vi "Get 2D Picture from Map.vi"(8 "error in (no error)":errorcluster, 11 "Grassfire in":refnum<class "Grassfire.lvclass">) -> (0 "error out":errorcluster, 2 "2D Picture":picture, 3 "Grassfire out":refnum<class "Grassfire.lvclass">)   [LabVIEW 2019, in "Grassfire.lvclass"]
uses:
  Grassfire.lvclass
  Grassfire.lvclass/Grassfire.ctl
  Address/Address.lvclass/Address.ctl
  Node/Node Value.lvclass/Node Value.ctl
  Node/Read Distance.vi
  Node/Read Node Type.vi
  Address/Read Row.vi
  Address/Read Column.vi
  Address/Address.lvclass
  Node/Node Value.lvclass
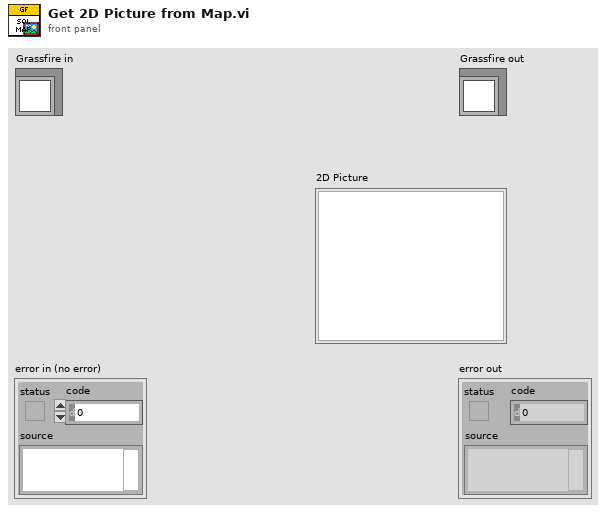
[diagram p1: front panel]
types:
  T1 = map{refnum<class "Address.lvclass">, refnum<class "Node Value.lvclass">}
  T2 = typedef "Picture Ring.lvclass/Node Type--enum.ctl" = enum16{"Empty", "Blocked", "Start", "End", "Path"}
  T3 = typedef "imagedata.ctl" = cluster{"image type":i32, "image depth":i32, "image":u8[], "mask":u8[], "colors":u32[], "Rectangle":cluster{"left":i16, "top":i16, "right":i16, "bottom":i16}}
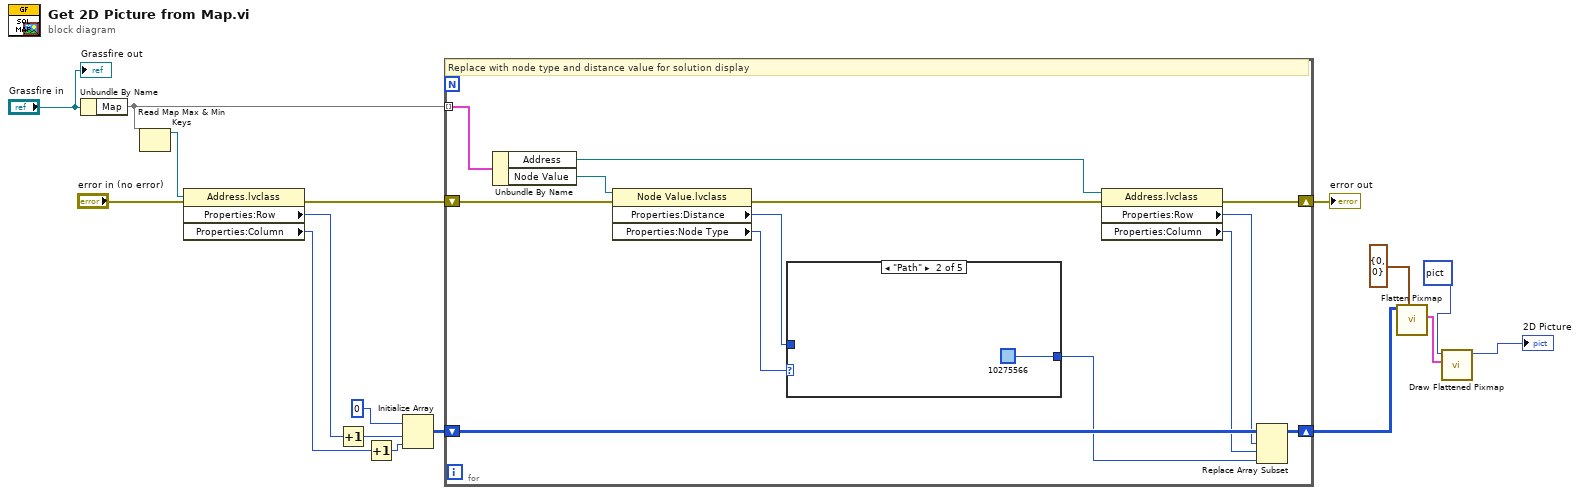
[diagram p0: block diagram]
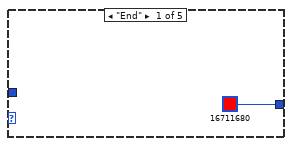
[diagram p2: hidden frame]
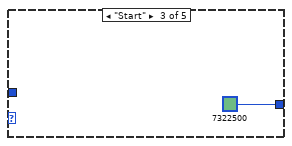
[diagram p3: hidden frame]
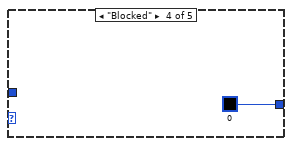
[diagram p4: hidden frame]
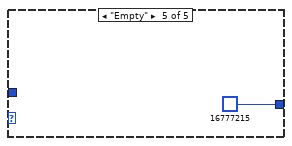
[diagram p5: hidden frame]
diagram:
  n1 = Unbundle By Name("Grassfire in") -> ("Map"=w11:T1)
  n2 = Read Map Max & Min Keys(11:w11) -> (3:w17:refnum<class "Address.lvclass">)  [unwired: 1 out]
  n3 = property class="Address.lvclass"(reference=w17, error in="error in (no error)") -> (error out=w8:errorcluster, "Properties:Row"=w16:i32, "Properties:Column"=w15:i32)  [unwired: 1 out]
  n4 = Increment(x=w16) -> (x+1=w14:i32)
  n5 = Increment(x=w15) -> (x+1=w13:i32)
  n6 = Initialize Array(u32 0, w14, w13) -> (w12:u32[][])
  n7 = for {
    shift-right: [w28] -> w2
    shift-left: w12 -> [w29]
    tunnel: w11 -> [w30] mode=indexing
    shift-right: [w21] -> w7
    shift-left: w8 -> [w23]
    # "Replace with node type and distance value for solution display"
    n8 = Unbundle By Name(w30) -> ("Address"=w27:refnum<class "Address.lvclass">, "Node Value"=w24:refnum<class "Node Value.lvclass">)
    n9 = property class="Node Value.lvclass"(reference=w24, error in=w23) -> (error out=w22:errorcluster, "Properties:Distance"=w20:i32, "Properties:Node Type"=w19:T2)  [unwired: 1 out]
    n10 = case shown="\"Path\"" w19 {
      tunnel: w20 -> [_ _ _ _ _]
      tunnel: [u32 16711680 ("Pen Color") u32 10275566 ("Pen Color") u32 7322500 ("Pen Color") u32 0 ("Pen Color") u32 16777215 ("Pen Color")] -> w18
      frame "End" {
      }
      frame "Path" {
      }
      frame "Start" {
      }
      frame "Blocked" {
      }
      frame "Empty" {
      }
    }
    n11 = property class="Address.lvclass"(reference=w27, error in=w22) -> (error out=w21:errorcluster, "Properties:Row"=w26:i32, "Properties:Column"=w25:i32)  [unwired: 1 out]
    n12 = Replace Array Subset(array=w29, new element=w18, index (row)=w26, index (col)=w25) -> (w28:u32[][])
  }
  "error out" <- w7
  n13 = call <vilib>:"Flatten Pixmap.vi"("top left"=cluster{"x":i16, "y":i16} {"x"=0, "y"=0}, "24-bit pixmap"=w2) -> ("image data"=w3:T3)  [unwired: 9 in]
  n14 = call <vilib>:"Draw Flattened Pixmap.vi"("image data"=w3, "picture"=picture data[5B]) -> ("new picture"=→"2D Picture":picture)  [unwired: 7 in]
  "Grassfire out" <- "Grassfire in"
